vi "GRIMMcontrollerVI.vi"(8 "error in (no error)":errorcluster) -> (0 "error out":errorcluster)   [LabVIEW 2013]
doc: "Use this template to build a VI to use as a subVI."
uses:
  <vilib>/Instr/_visa.llb/VISA Configure Serial Port (Instr).vi
panel:
  out "Number of Particles":i32[](array[numeric])
  in  "error in (no error) 2":errorcluster
  in  "Set Interval Time Button":bool
  in  "Interval Time":T1(ring)
  out "read buffer":string
  in  "Stop GRIMM Measurement":bool
  in  "Start GRIMM Measurement":bool
  in  "stop":bool
  in  "GRIMM Com Port":refnum<visa-resource-name>="COM16"
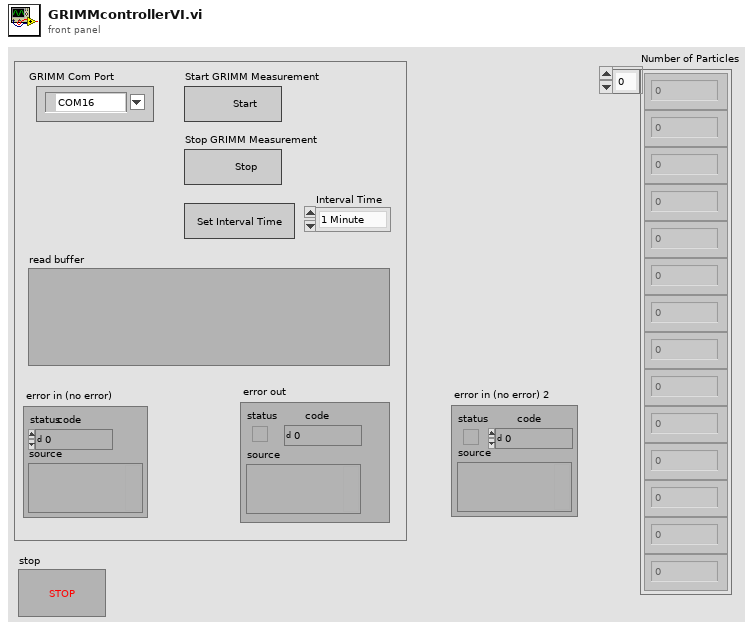
[diagram p1: front panel]
types:
  T1 = enum16{"1 Minute", "5 Mintues", "10 Minutes", "15 Minutes", "30 Minutes", "60 Minutes", "6 Seconds", "3 Seconds", "2 Seconds", "1 Second"}
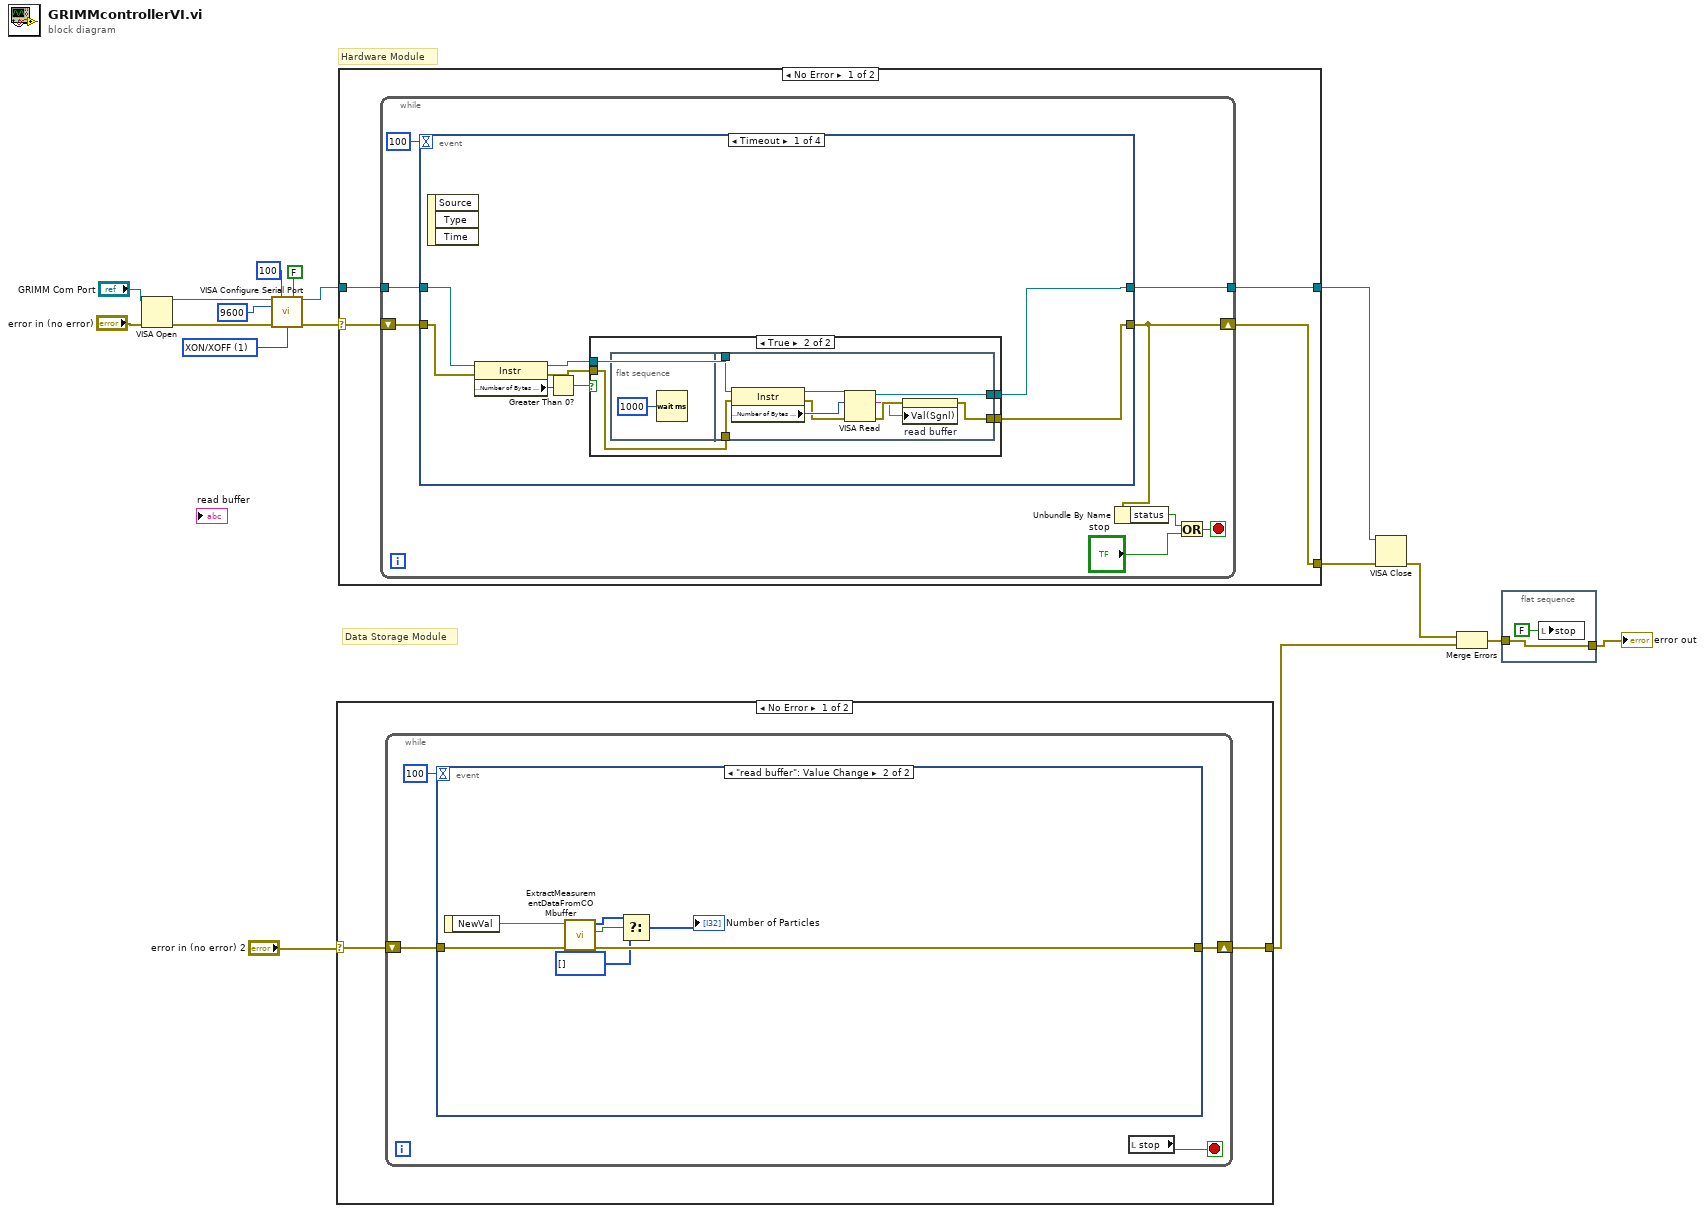
[diagram p0: block diagram]
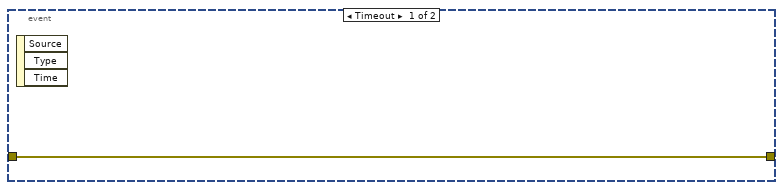
[diagram p2: hidden frame]
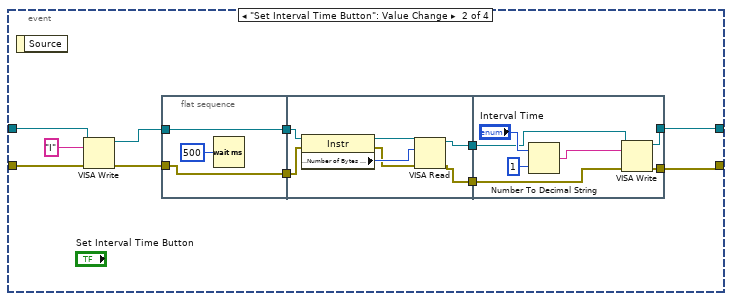
[diagram p5: hidden frame]
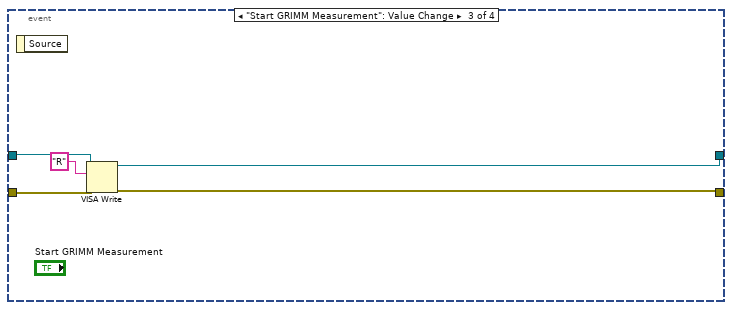
[diagram p6: hidden frame]
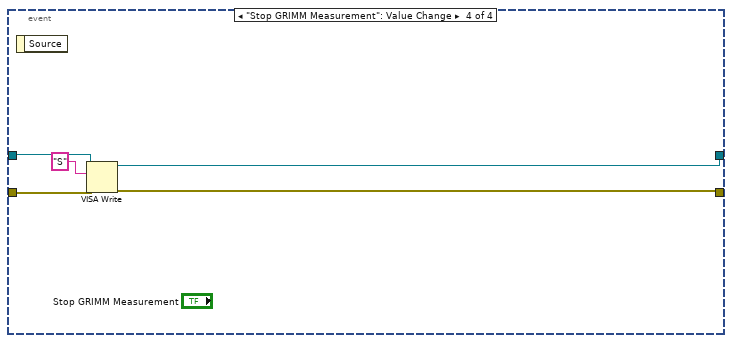
[diagram p7: hidden frame]
diagram:
  w10 = u16 1 items=["None", "XON/XOFF", "RTS/CTS", "XON/XOFF & RTS/CTS", "DTR/DSR", "XON/XOFF & DTR/DSR"] ("flow control (0:none)")
  # "Data Storage Module"
  # "Hardware Module"
  n1 = VISA Open(error in (no error)="error in (no error)", VISA resource name="GRIMM Com Port") -> (VISA resource name=w17:refnum<visa-resource-name>, error out=w16:errorcluster)  [unwired: 3 in]
  n2 = call-poly "VISA Configure Serial Port"("VISA resource name"=w17, "timeout (10sec)"=u32 100, "Enable Termination\nChar (T)"=FALSE ("Enable Termination\nChar (T)"), "baud rate (9600)"=u32 9600, "error in (no error)"=w16, "flow control (0:none)"=w10) -> ("VISA resource name out"=w7:refnum<visa-resource-name>, "error out"=w9:errorcluster)  [unwired: 8 in]
  n3 = case shown="No Error" "error in (no error) 2" {
    selector: "error in (no error) 2" -> [w19 w32]
    tunnel: [w18 w32] -> w4
    frame No Error {
      n4 = while {
        shift-right: [w21] -> w18
        shift-left: w19 -> [w22]
        stop <- w23 stop-if-true
        n5 = event shown="[1] \"read buffer\": Value Change" {
          selector: _ -> [_ _]
          dyn-events: _ -> [_ _]
          timeout: 100 -> [_ _]
          tunnel: w22 -> [w24 w30]
          tunnel: [w24 w29] -> w21
          event Timeout {
            n6 = event-data() -> ()  [unwired: 1 in, 3 out]
          }
          event "read buffer": Value Change {
            n7 = event-data() -> ("NewVal"=w31:string)  [unwired: 1 in]
            n8 = call "ExtractMeasurementDataFromCOMbuffer.vi"("error in (no error)"=w30, "Input OPC data"=w31) -> ("error out"=w29:errorcluster, "Valid Data"=w28:bool, "Output Number of Particles per 100 CC"=w27:i32[])  [unwired: 7 in]
            n9 = Select(t=w27, s=w28, f=i32[] []) -> (s? t:f=→"Number of Particles":i32[])
          }
        }
        n10 = local read "stop"() -> (w23:bool)
      }
    }
    frame Error {
    }
  }
  n11 = case shown="No Error" w9 {
    selector: w9 -> [w35 w108]
    tunnel: [w34 w108] -> w8
    tunnel: w7 -> [w36 w107]
    tunnel: [w33 w107] -> w6
    frame No Error {
      n12 = while {
        tunnel: w36 -> [w43]
        tunnel: [w42] -> w33
        shift-right: [w41] -> w34
        shift-left: w35 -> [w44]
        stop <- w38 stop-if-true
        n13 = event shown="[0] Timeout" {
          selector: _ -> [_ _ _ _]
          dyn-events: _ -> [_ _ _ _]
          timeout: 100 -> [_ _ _ _]
          tunnel: w44 -> [w48 w79 w99 w104]
          tunnel: [w45 w71 w98 w103] -> w41
          tunnel: [w46 w70 w97 w102] -> w42
          tunnel: w43 -> [w52 w78 w100 w105]
          event Timeout {
            n14 = event-data() -> ()  [unwired: 1 in, 3 out]
            n15 = property class="Instr"(reference=w52, error in=w48) -> (reference out=w49:refnum<visa-resource-name>, error out=w47:errorcluster, "Serial Settings:Number of Bytes at Serial Port"=w50:u32)
            n16 = Greater Than 0?(x=w50) -> (x > 0?=w51:bool)
            n17 = case shown="True" w51 {
              tunnel: w49 -> [w53 w58]
              tunnel: w47 -> [w54 w57]
              tunnel: [w53 w56] -> w46
              tunnel: [w54 w55] -> w45
              frame False {
              }
              frame True {
                n18 = flat-sequence {
                  tunnel: w58 -> [w68]
                  tunnel: w57 -> [w65]
                  tunnel: [w63] -> w56
                  tunnel: [w61] -> w55
                  frame #0 {
                    n19 = Wait (ms)(milliseconds to wait=u32 1000) -> ()  [unwired: 1 out]
                  }
                  frame #1 {
                    n20 = property class="Instr"(reference=w68, error in=w65) -> (reference out=w67:refnum<visa-resource-name>, error out=w64:errorcluster, "Serial Settings:Number of Bytes at Serial Port"=w66:u32)
                    n21 = VISA Read(VISA resource name=w67, byte count=w66, error in (no error)=w64) -> (VISA resource name out=w63:refnum<visa-resource-name>, read buffer=w60:string, error out=w62:errorcluster)  [unwired: 1 out]
                    n22 = property on="read buffer" class="Str"(error in=w62, "Val(Sgnl)"=w60) -> (error out=w61:errorcluster)  [unwired: 1 in, 1 out]
                  }
                }
              }
            }
          }
          event "Set Interval Time Button": Value Change {
            n23 = event-data() -> ()  [unwired: 1 in, 1 out]
            n24 = VISA Write(VISA resource name=w78, write buffer="I" ("string"), error in (no error)=w79) -> (VISA resource name out=w76:refnum<visa-resource-name>, error out=w75:errorcluster)  [unwired: 1 out]
            n25 = flat-sequence {
              tunnel: w76 -> [w81]
              tunnel: w75 -> [w80]
              tunnel: [w81] -> w74
              tunnel: [w80] -> w69
              tunnel: w74 -> [w86]
              tunnel: [w85] -> w73
              tunnel: [w84] -> w72
              tunnel: w69 -> [w83]
              tunnel: w73 -> [w94]
              tunnel: w72 -> [w93]
              tunnel: [w92] -> w71
              tunnel: [w91] -> w70
              frame #0 {
                n26 = Wait (ms)(milliseconds to wait=u32 500) -> ()  [unwired: 1 out]
              }
              frame #1 {
                n27 = property class="Instr"(reference=w86, error in=w83) -> (reference out=w89:refnum<visa-resource-name>, error out=w87:errorcluster, "Serial Settings:Number of Bytes at Serial Port"=w88:u32)
                n28 = VISA Read(VISA resource name=w89, byte count=w88, error in (no error)=w87) -> (VISA resource name out=w85:refnum<visa-resource-name>, error out=w84:errorcluster)  [unwired: 2 out]
              }
              frame #2 {
                n29 = Number To Decimal String(number="Interval Time", width (-)=i16 1) -> (decimal integer string=w90:string)
                n30 = VISA Write(VISA resource name=w94, write buffer=w90, error in (no error)=w93) -> (VISA resource name out=w91:refnum<visa-resource-name>, error out=w92:errorcluster)  [unwired: 1 out]
              }
            }
          }
          event "Start GRIMM Measurement": Value Change {
            n31 = event-data() -> ()  [unwired: 1 in, 1 out]
            n32 = VISA Write(VISA resource name=w100, write buffer="R", error in (no error)=w99) -> (VISA resource name out=w97:refnum<visa-resource-name>, error out=w98:errorcluster)  [unwired: 1 out]
          }
          event "Stop GRIMM Measurement": Value Change {
            n33 = event-data() -> ()  [unwired: 1 in, 1 out]
            n34 = VISA Write(VISA resource name=w105, write buffer="S", error in (no error)=w104) -> (VISA resource name out=w102:refnum<visa-resource-name>, error out=w103:errorcluster)  [unwired: 1 out]
          }
        }
        n35 = Unbundle By Name(w41) -> ("status"=w40:bool)
        n36 = Or(x=w40, y="stop") -> (x .or. y?=w38:bool)
      }
    }
    frame Error {
    }
  }
  n37 = VISA Close(VISA resource name=w6, error in (no error)=w8) -> (error out=w3:errorcluster)
  n38 = Merge Errors(w3, w4) -> (w2:errorcluster)
  n39 = flat-sequence {
    tunnel: w2 -> [w109]
    tunnel: [w109] -> w1
    frame #0 {
      n40 = local write "stop"(FALSE ("stop")) -> ()
    }
  }
  "error out" <- w1
